vi "Setup FC2 ILC.vi"(8 "error in (no error)":errorcluster, 10 "Model in":refnum<class "Model.lvclass">, 11 "Boot Loader in":refnum<class "Boot Loader.lvclass">) -> (0 "error out":errorcluster, 2 "Model out":refnum<class "Model.lvclass">, 3 "Boot Loader out":refnum<class "Boot Loader.lvclass">)   [LabVIEW 2015, in "Boot Loader.lvclass"]
uses:
  Boot Loader.lvclass
  Model/Model.lvclass
  <userlib>/Common/SerialProtocols/SerialProtocolFactory/SerialProtocolFactory/SerialProtocolFactory.lvclass
  <userlib>/Common/SerialProtocols/SerialCommunicator/SerialCommunicator.lvclass
  <userlib>/Common/ILC/ILC/ILC.lvclass
  <userlib>/Common/SerialProtocols/SerialCommunicator/SerialCommunicator.lvclass/SerialCommunicator.ctl
  <userlib>/Common/ILC/ILC/ILC.lvclass/ILC.ctl
  Model/Model.lvclass/Model.ctl
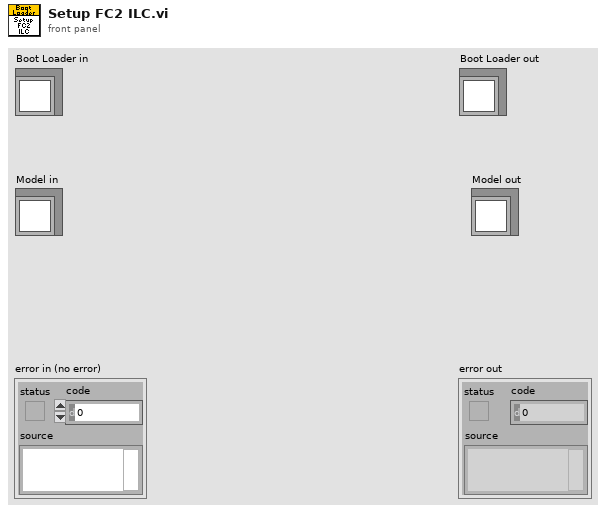
[diagram p1: front panel]
types:
  T1 = typedef "ILCCommon.lvlib/ILCConfiguration.lvlib/Serial.ctl" = cluster{"Serial":T2}
  T2 = typedef "SerialProtocols.lvlib/SerialConfig.ctl" = cluster{"Serial Protocol":T3, "Protocol Parameters":T4, "Serial Message Parameters":T5}
  T3 = typedef "SerialProtocols.lvlib/SerialProtocol.ctl" = enum16{"RS232", "RS485", "SerialSimulator"}
  T4 = typedef "SerialProtocols.lvlib/ProtocolParameters.ctl" = cluster{"VISA resource name":refnum<visa-resource-name>, "Baud Rate":u32, "Data Bits":u16, "Parity":enum16{"None", "Odd", "Even", "Mark", "Space"}, "Flow Control":u16, "Stop Bits":u16, "Timeout (ms)":u32}
  T5 = typedef "SerialProtocols.lvlib/SerialMessageParameters.ctl" = cluster{"Byte Count":u32, "Enable Termination Character":bool, "Termination Char":u8}
  T6 = typedef "ILCCommon.lvlib/ILCConfiguration.lvlib/ADC.ctl" = cluster{"Reference Voltage Vref":dbl[unit], "Nominal Input Range in Counts":u32, "Preamplifier Gain":u8, "Conversion Settling Cycles":u16}
  T7 = typedef "ILCCommon.lvlib/ILCTypedefs.lvlib/ADC Settings.ctl" = cluster{"Input Channels":T8, "Scan Rate (Hz) ":T9, "PGA Gain Coefficient":u8}
  T8 = typedef "ILCCommon.lvlib/ILCConfiguration.lvlib/Input Channels.ctl" = enum16{"Channel 0", "3 Channels", "5 Channels"}
  T9 = typedef "ILCCommon.lvlib/ILCConfiguration.lvlib/Scan Rates.ctl" = enum16{"50", "60", "100", "120", "200", "240", "300", "400", "480", "600", "1200", "2400", "4800"}
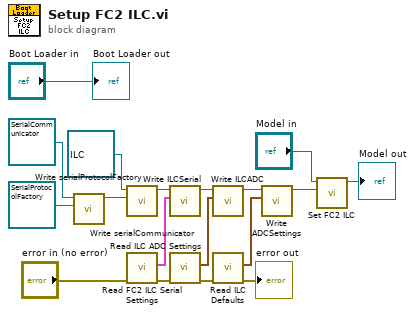
[diagram p0: block diagram]
diagram:
  n1 = call <userlib>:"Write serialProtocolFactory.vi"("serialProtocolFactory"=refnum<class "SerialProtocolFactory.lvclass"> refnum ("SerialCommFactory.lvclass"), "SerialCommunicator in"=refnum<class "SerialCommunicator.lvclass"> refnum ("SerialProtocols.lvlib:SerialCommunicator.lvclass")) -> ("SerialCommunicator out"=w15:refnum<class "SerialCommunicator.lvclass">)  [unwired: 9 in]
  n2 = call <userlib>:"Write serialCommunicator.vi"("serialCommunicator"=w15, "ILC in"=refnum<class "ILC.lvclass"> refnum ("ILCCommon.lvlib:ILC.lvclass")) -> ("ILC out"=w11:refnum<class "ILC.lvclass">)  [unwired: 9 in]
  n3 = call "Read FC2 ILC Serial Settings.vi"("error in (no error)"="error in (no error)") -> ("error out"=w7:errorcluster, "ILC Serial Settings"=w10:T1)  [unwired: 8 in, 1 out]
  n4 = call <userlib>:"Write ILCSerial.vi"("ILC Serial"=w10, "ILC in"=w11) -> ("ILC out"=w8:refnum<class "ILC.lvclass">)  [unwired: 9 in]
  n5 = call "Read ILC ADC Settings.vi"("error in (no error)"=w7) -> ("error out"=w4:errorcluster, "ILC ADC Settings"=w9:T6)  [unwired: 8 in, 1 out]
  n6 = call <userlib>:"Write ILCADC.vi"("ILC ADC"=w9, "ILC in"=w8) -> ("ILC out"=w5:refnum<class "ILC.lvclass">)  [unwired: 9 in]
  n7 = call "Read ILC Defaults.vi"("error in (no error)"=w4) -> ("error out"=→"error out":errorcluster, "ILC Default Settings"=w6:T7)  [unwired: 8 in, 1 out]
  n8 = call <userlib>:"Write ADCSettings.vi"("ADC Settings"=w6, "ILC in"=w5) -> ("ILC out"=w3:refnum<class "ILC.lvclass">)  [unwired: 9 in]
  n9 = call "Set FC2 ILC.vi"("FC2ILC"=w3, "Model in"="Model in") -> ("Model out"=→"Model out":refnum<class "Model.lvclass">)  [unwired: 9 in]
  "Boot Loader out" <- "Boot Loader in"
